vi "log_template.vi"(4 "接收报文":string="URL=", 6 "a:Success":string, 7 "URL":string="URL=", 8 "StartTime":string, 10 "发送报文":string) -> ()   [LabVIEW 2020]
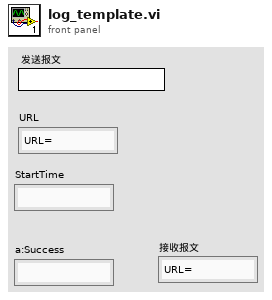
[diagram p1: front panel]
types:
  T1 = enum16{"open", "replace", "create", "open or create", "replace or create", "replace or create with confirmation"}
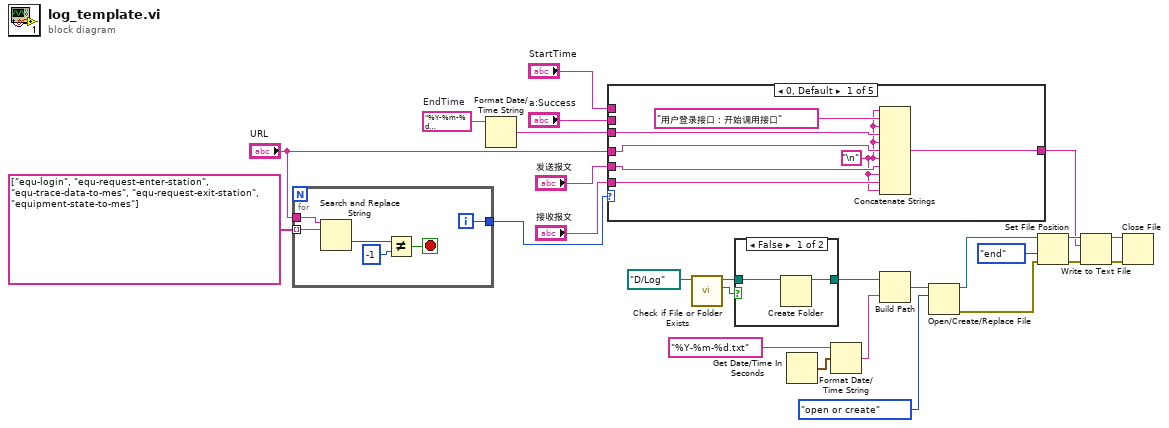
[diagram p0: block diagram]
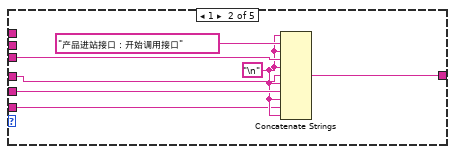
[diagram p2: hidden frame]
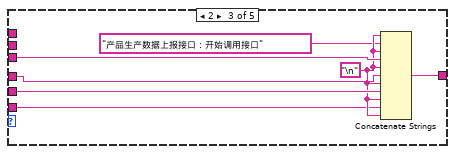
[diagram p3: hidden frame]
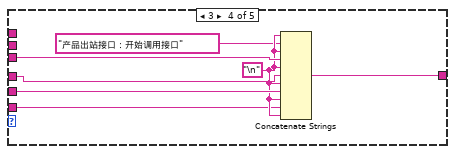
[diagram p4: hidden frame]
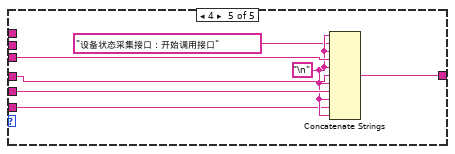
[diagram p5: hidden frame]
diagram:
  w15 = "%Y-%m-%d %H:%M:%S%3u-->"  # EndTime
  n1 = for {
    tunnel: string[] ["equ-login", "equ-request-enter-station", "equ-trace-data-to-mes", "equ-request-exit-station", "equipment-state-to-mes"] ("字符串数组") -> [w28] mode=indexing
    tunnel: "URL" -> [w32]
    tunnel: [w27] -> w18
    i -> [w27]
    stop <- w29 stop-if-true
    n2 = Search and Replace String(input string=w32, search string=w28) -> (offset past replacement=w30:i32)  [unwired: 6 in, 3 out]
    n3 = Not Equal?(x=w30, y=-1) -> (x != y?=w29:bool)
  }
  n4 = Format Date/Time String(time format string (%c)=w15) -> (date/time string=w14:string)  [unwired: 2 in]
  n5 = case shown="0, Default" w18 {
    tunnel: "发送报文" -> [w38 w45 w52 w59 w66]
    tunnel: "StartTime" -> [_ _ _ _ _]
    tunnel: w14 -> [w36 w43 w51 w58 w65]
    tunnel: "a:Success" -> [_ _ _ _ _]
    tunnel: "接收报文" -> [w37 w40 w48 w55 w62]
    tunnel: [w39 w46 w53 w60 w67] -> w2
    tunnel: "URL" -> [w35 w41 w49 w56 w63]
    frame 0, Default {
      w33 = "\n"
      n6 = Concatenate Strings(w33, "用户登录接口：开始调用接口", w33, w36, w33, w35, w33, w38, w33, w37, w33) -> (w39:string)
    }
    frame 1 {
      w42 = "\n"
      n7 = Concatenate Strings(w42, "产品进站接口：开始调用接口", w42, w43, w42, w41, w42, w45, w42, w40, w42) -> (w46:string)
    }
    frame 2 {
      w50 = "\n"
      n8 = Concatenate Strings(w50, "产品生产数据上报接口：开始调用接口", w50, w51, w50, w49, w50, w52, w50, w48, w50) -> (w53:string)
    }
    frame 3 {
      w57 = "\n"
      n9 = Concatenate Strings(w57, "产品出站接口：开始调用接口", w57, w58, w57, w56, w57, w59, w57, w55, w57) -> (w60:string)
    }
    frame 4 {
      w64 = "\n"
      n10 = Concatenate Strings(w64, "设备状态采集接口：开始调用接口", w64, w65, w64, w63, w64, w66, w64, w62, w64) -> (w67:string)
    }
  }
  n11 = call <vilib>:"Check if File or Folder Exists.vi"("path"=path "D:/Log" ("路径")) -> ("file or folder exists?"=w24:bool, "dup path"=w25:path)  [unwired: 8 in, 1 out]
  n12 = case shown="False" w24 {
    tunnel: w25 -> [w69 w70]
    tunnel: [w68 w70] -> w22
    frame False {
      n13 = Create Folder(path (use dialog)=w69) -> (created path=w68:path)  [unwired: 2 in, 2 out]
    }
    frame True {
    }
  }
  n14 = Get Date/Time In Seconds() -> (seconds since 1Jan1904=w20:timestamp)
  n15 = Format Date/Time String(time format string (%c)="%Y-%m-%d.txt" ("时间格式字符串(%c)"), seconds (now)=w20) -> (date/time string=w19:string)  [unwired: 1 in]
  n16 = Build Path(base path=w22, name or relative path=w19) -> (appended path=w26:path)
  n17 = Open/Create/Replace File(file path (use dialog)=w26, operation (0:open)=T1."open or create" ("操作(0:open)")) -> (refnum out=w8:refnum<file>, error out=w9:errorcluster)  [unwired: 4 in, 1 out]
  n18 = Set File Position(refnum=w8, from (0:start)=enum16{"start", "end", "current"}."end" ("自（0:起始）"), error in=w9) -> (refnum out=w10:refnum<file>, error out=w11:errorcluster)  [unwired: 1 in]
  n19 = Write to Text File(file (use dialog)=w10, text=w2, error in=w11) -> (refnum out=w7:refnum<file>, error out=w6:errorcluster)  [unwired: 1 in, 1 out]
  n20 = Close File(refnum=w7, error in=w6) -> ()  [unwired: 2 out]
